vi "Drive Controller.vi"(8 "error in":errorcluster) -> ()   [LabVIEW 2018]
doc: "This VI executes continuously carrying out the current operation and responding to updates or new operation requests. It will often contain the timing or control code that is difficult to place directly in TeleOp. This VI generally opens all sensors and motors and isolates the rest of the robot code from knowing implementation details of how the operations are carried out."
uses:
  Drive Setpoints.ctl
  Drive Operations.ctl
  <vilib>/Rock Robotics/WPI/Solenoid/WPI_SolenoidChannel.ctl
  <vilib>/Rock Robotics/WPI/SafetyOutput/WPI_SafetyOutputConfigMenu.ctl
  <vilib>/Rock Robotics/WPI/ThirdParty/Phoenix-LabVIEW/Motor Controller/Controls/CTRE_Phoenix_MotorControl_NeutralMode.ctl
  <vilib>/Rock Robotics/WPI/ThirdParty/Phoenix-LabVIEW/Motor Controller/Controls/CTRE_Phoenix_MotorControl_FeedbackDevice.ctl
  <vilib>/Rock Robotics/WPI/ThirdParty/Phoenix-LabVIEW/Motor Controller/Controls/CTRE_Phoenix_MotorControl_ControlMode.ctl
  <vilib>/Rock Robotics/WPI/ThirdParty/Phoenix-LabVIEW/Motor Controller/Controls/CTRE_Phoenix_MotorControl_StatusFrameEnhanced.ctl
  <vilib>/Rock Robotics/WPI/Solenoid/WPI_SolenoidValue.ctl
  <vilib>/Rock Robotics/WPI/Solenoid/WPI_SolenoidOpenSingle.vi
  <vilib>/Rock Robotics/WPI/Solenoid/WPI_SolenoidSetEnum.vi
  <vilib>/Rock Robotics/WPI/Utilities/WPI_GetSetVariantRefNum.vi
  <vilib>/Rock Robotics/WPI/RobotDrive/WPI_RobotDriveMecanumDrive_Cartesian.vi
  <vilib>/Rock Robotics/WPI/ThirdParty/Phoenix-LabVIEW/Motor Controller/Get/CTRE_Phoenix_MotorController_GetQuadratureData.vi
panel:
  out "Current\nCmd":string
  # ".578"
  # "Tip: It may be helpful to observe inputs and sensor values.\nYou may also want to display tuning or debugging controls."
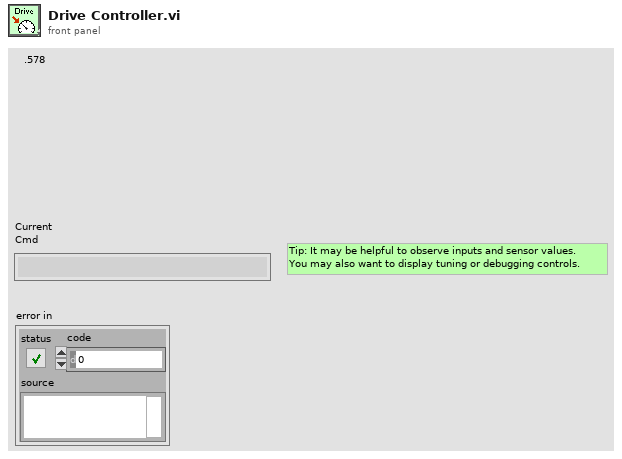
[diagram p1: front panel]
types:
  T1 = typedef "CTRE_Phoenix_MotorControl_StatusFrameEnhanced.ctl" = u16
  T2 = typedef "WPI_SolenoidChannel.ctl" = enum8{"Solenoid 0", "Solenoid 1", "Solenoid 2", "Solenoid 3", "Solenoid 4", "Solenoid 5", "Solenoid 6", "Solenoid 7", "Invalid"}
  T3 = typedef "CTRE_Phoenix_MotorControl_FeedbackDevice.ctl" = i8
  T4 = typedef "CTRE_Phoenix_MotorControl_NeutralMode.ctl" = enum8{"EEPROMSetting", "Override to Coast", "Override to Brake"}
  T5 = typedef "CTRE_Phoenix_MotorControl_ControlMode.ctl" = u16
  T6 = typedef "WPI_SafetyOutputConfigMenu.ctl" = enum16{"Enable", "Disable"}
  T7 = typedef "Drive Setpoints.ctl" = cluster{"Operation":T8, "X Setpoint":dbl, "Y Setpoint":dbl, "Duration":dbl, "Z Setpoint":dbl, "Tracks":bool, "Gyro":dbl, "POV":i16, "Distance(feet)":dbl, "AutoTrack Toggle":bool, "Collsision Detection":bool, "Reset Encoder":bool, "MP File Name":string}
  T8 = typedef "Drive Operations.ctl" = enum16{"Reserve", "Read Current", "Reset Motors VBus", "Motion Profile run", "Immediate Robot Centric", "Drive for Time Robot Centric", "Immediate Field Centric", "Drive For Time Field Centric", "Button Adjust", "Set Motors Motion Profile", "Reset Encoders", "Motion Profile Enable", "Drive for Distance"}
  T9 = typedef "WPI_MotorControlDeviceRef.ctl" = cluster{"DeviceStatus":errorcluster, "Type":T10, "PWM":cluster{"PWM Channel":T11, "DeadBand":T12}, "CAN":cluster{"Device Number":u8, "SetOutput VI Ref":variant, "GetOutput VI Ref":variant, "Enable VI Ref":variant, "Disable VI Ref":variant, "Data":variant}, "Invert":bool, "DIO PWM":cluster{"PWM \"Enable\" Channel":T11, "DIOChannel":T13, "PWM Rate":dbl}}
  T10 = typedef "WPI_MotorControlType.ctl" = enum16{"PWM", "CAN", "DIO PWM"}
  T11 = typedef "FPGA_DIOPWMChannel.ctl" = enum8{"PWM 0", "PWM 1", "PWM 2", "PWM 3", "PWM 4", "PWM 5", "PWM 6", "PWM 7", "PWM 8", "PWM 9", "PWM MXP 0", "PWM MXP 1", "PWM MXP 2", "PWM MXP 3", "PWM MXP 4", "PWM MXP 5", "PWM MXP 6", "PWM MXP 7", "PWM MXP 8", "PWM MXP 9", "Invalid"}
  T12 = typedef "WPI_PWMDeadband.ctl" = cluster{"Name":string, "maxPositivePwm":i32, "minPositivePwm":i32, "centerPwm":i32, "maxNegativePwm":i32, "minNegativePwm":i32, "angularRange":u16}
  T13 = typedef "FPGA_DIOChannel.ctl" = enum8{"DIO 0", "DIO 1", "DIO 2", "DIO 3", "DIO 4", "DIO 5", "DIO 6", "DIO 7", "DIO 8", "DIO 9", "DIO MXP 0", "DIO MXP 1", "DIO MXP 2", "DIO MXP 3", "DIO MXP 4", "DIO MXP 5", "DIO MXP 6", "DIO MXP 7", "DIO MXP 8", "DIO MXP 9", "DIO MXP 10", "DIO MXP 11", "DIO MXP 12", "DIO MXP 13", "DIO MXP 14", "DIO MXP 15", "SPI Port CS1", "SPI Port CS2", "SPI Port CS3", "SPI Port MISO", "SPI Port MOSI", "Invalid"}
  T14 = typedef "WPI_RobotDriveDevRef.ctl" = cluster{"DevStatus":errorcluster, "Motors[]":T9[], "Square Inputs":bool, "Max Output":dbl}
  T15 = typedef "WPI_SolenoidDevRef.ctl" = cluster{"DevStatus":errorcluster, "Pneumatics Control Module":u8, "Forward Solenoid Channel":T2, "Reverse Solenoid Channel":T2}
  T16 = typedef "Command Status Info.ctl" = cluster{"Name":string, "Status":T17, "notifier out":T18}
  T17 = typedef "Completion Status.ctl" = enum16{"Successful", "Aborted", "Incomplete"}
  T18 = typedef "Completion Notifier.ctl" = refnum<notifier>
  T19 = cluster{"SubSystem Data":T7, cluster{"Start Time (ms)":u32, "Iterations":i32}, cluster{"Command Info":T16, "Description":string, "SubSystem Data":T7, "notifier out":refnum<notifier>, "Subsystem Name":string}}
  T20 = cluster{"proportional gain (Kc)":dbl, "integral time (Ti, min)":dbl, "derivative time (Td, min)":dbl}
  T21 = typedef "WPI_SolenoidValue.ctl" = enum16{"Off", "On", "Forward", "Reverse"}
  T22 = cluster{"SubSystem Data":T7, cluster{"Start Time (ms)":u32, "Iterations":i32}, "Default Command Arguments":cluster{"Command Info":T16, "Description":string, "SubSystem Data":T7, "notifier out":refnum<notifier>, "Subsystem Name":string}}
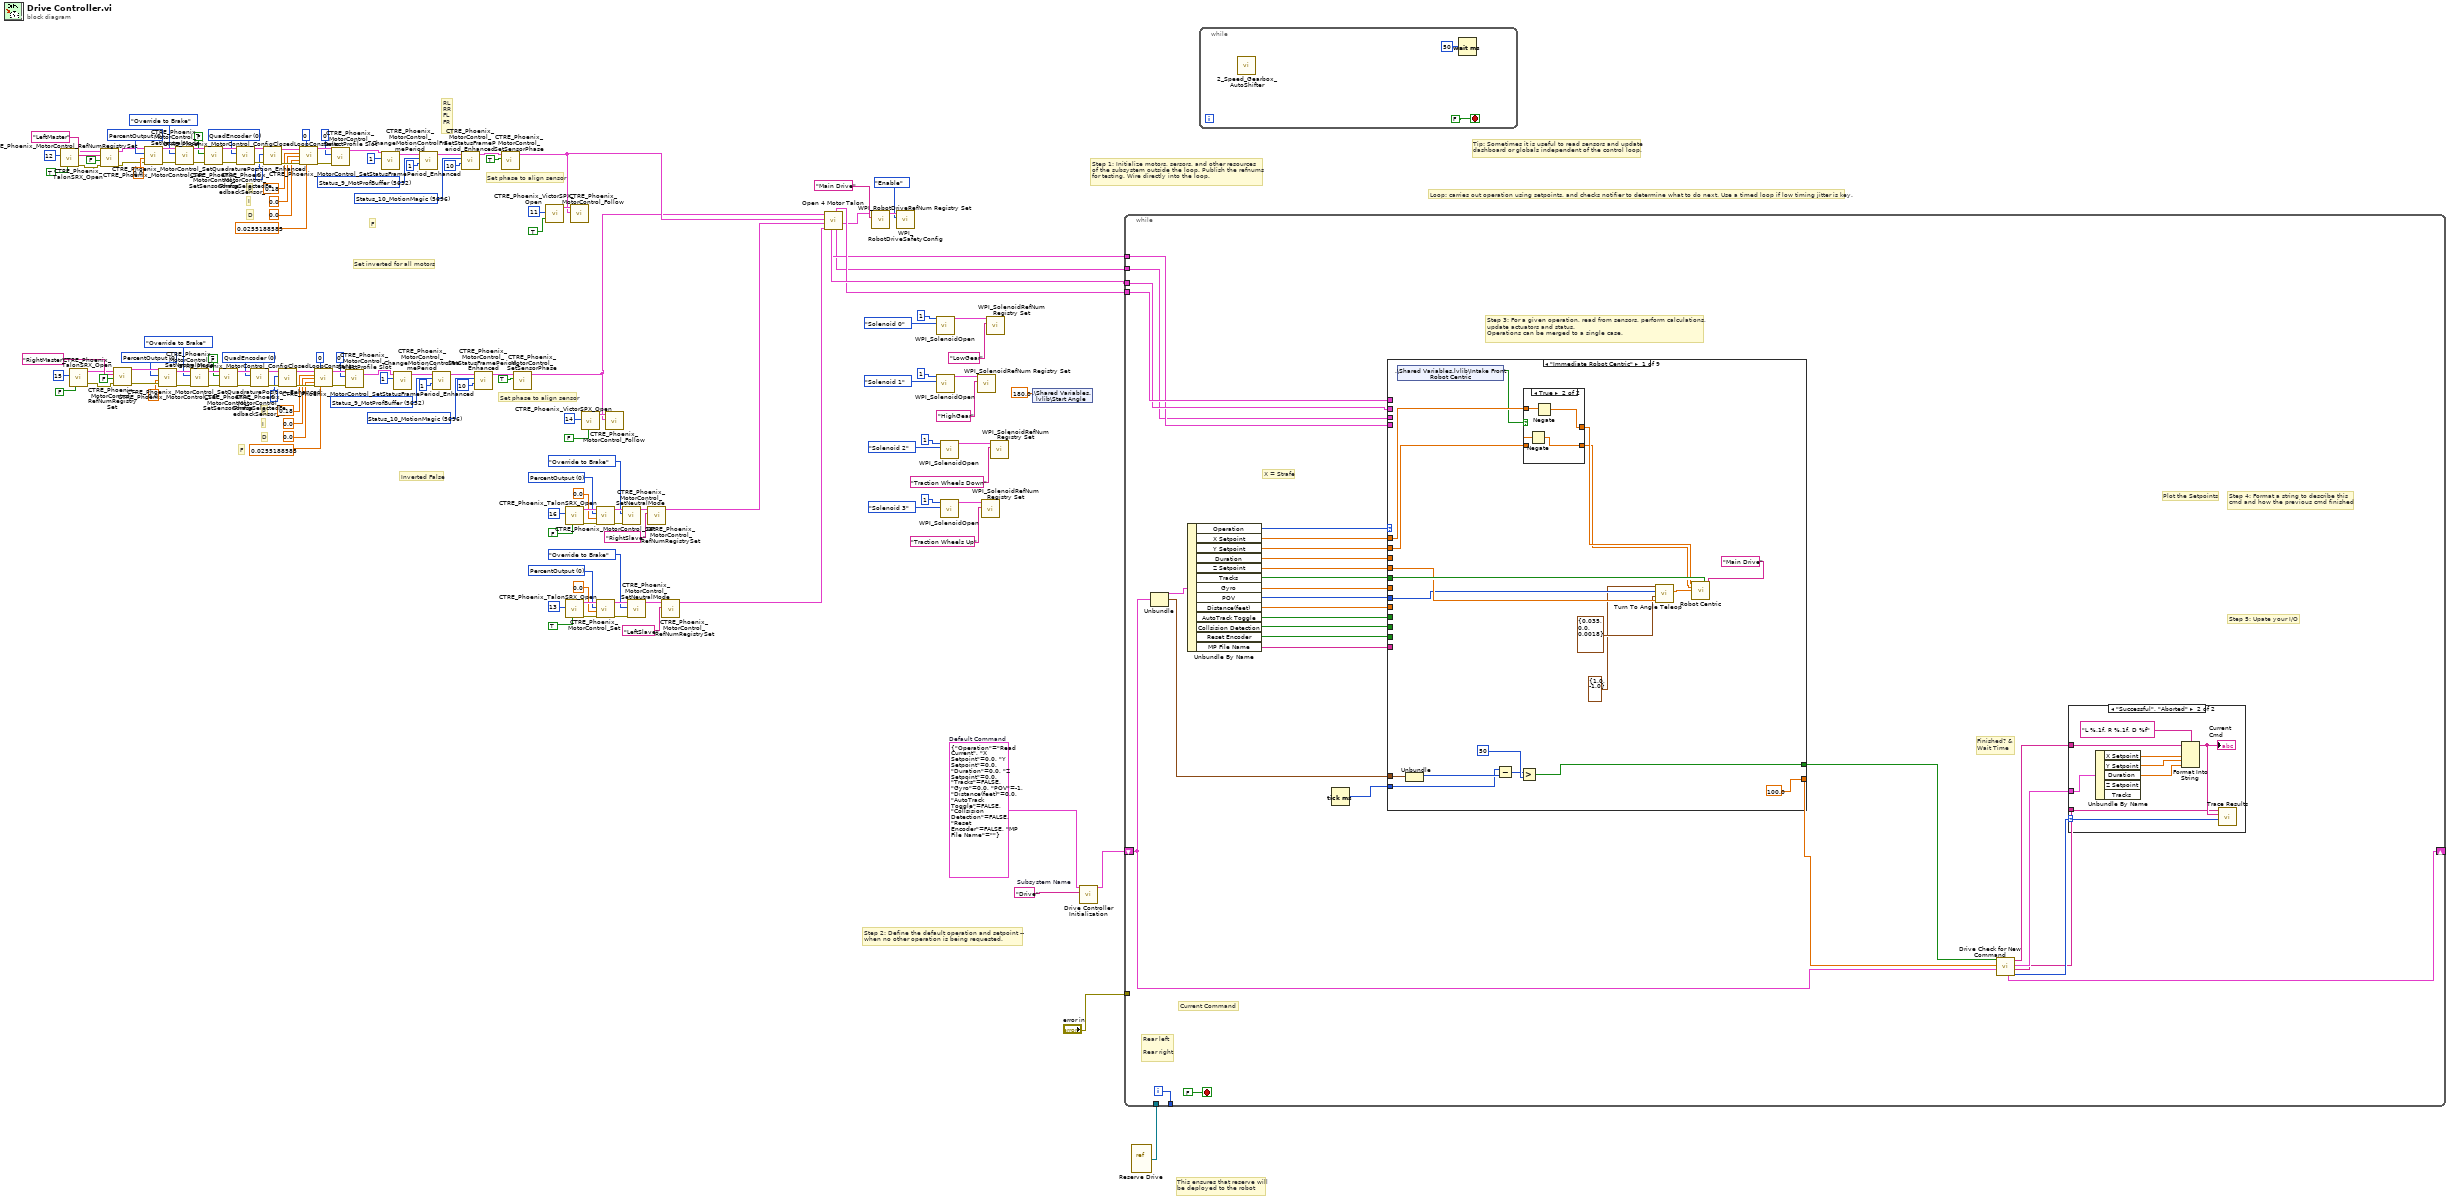
[diagram p0: block diagram]
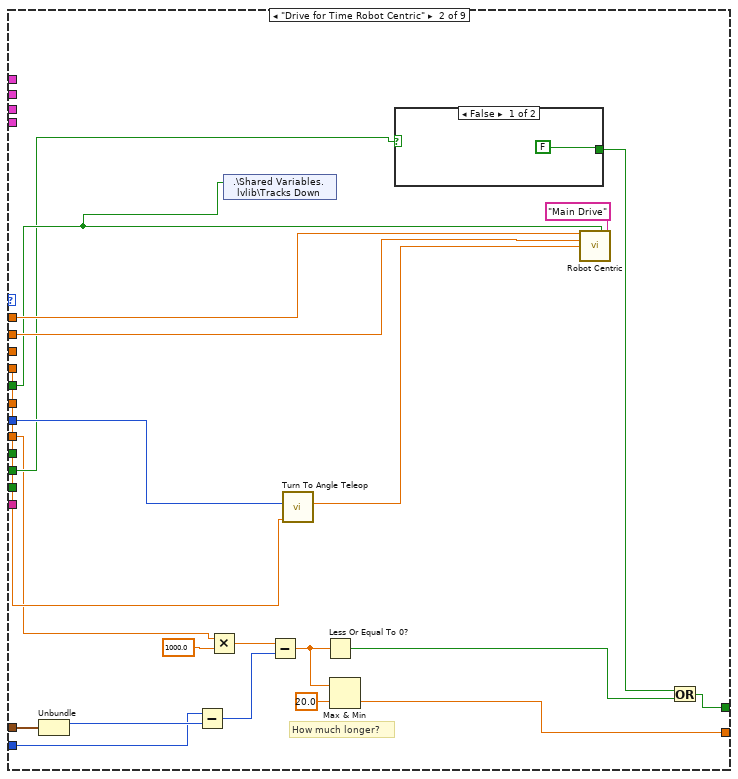
[diagram p4: hidden frame]
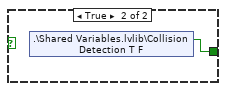
[diagram p5: hidden frame]
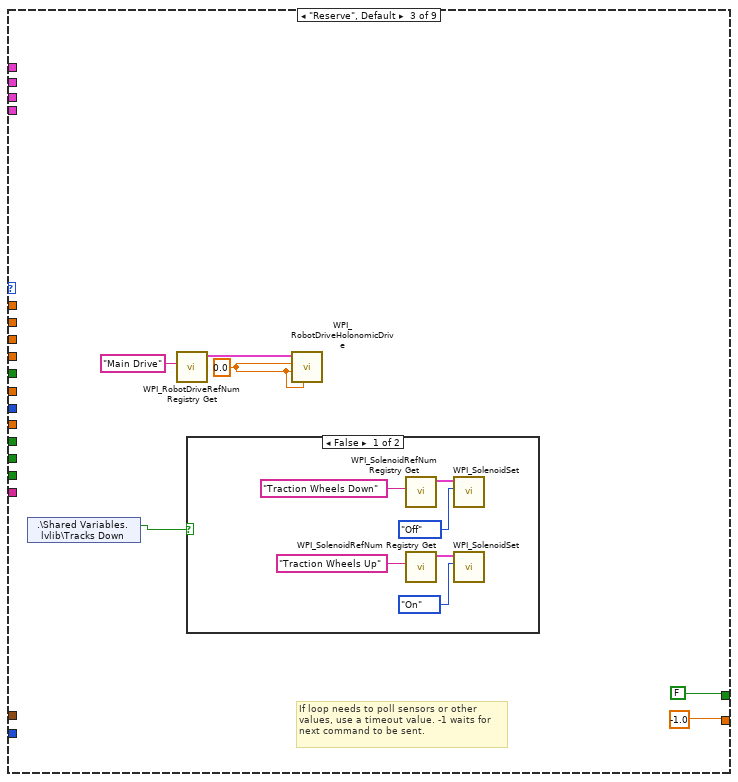
[diagram p6: hidden frame]
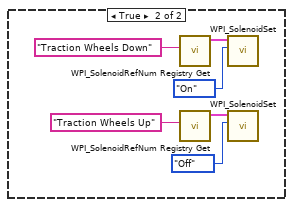
[diagram p7: hidden frame]
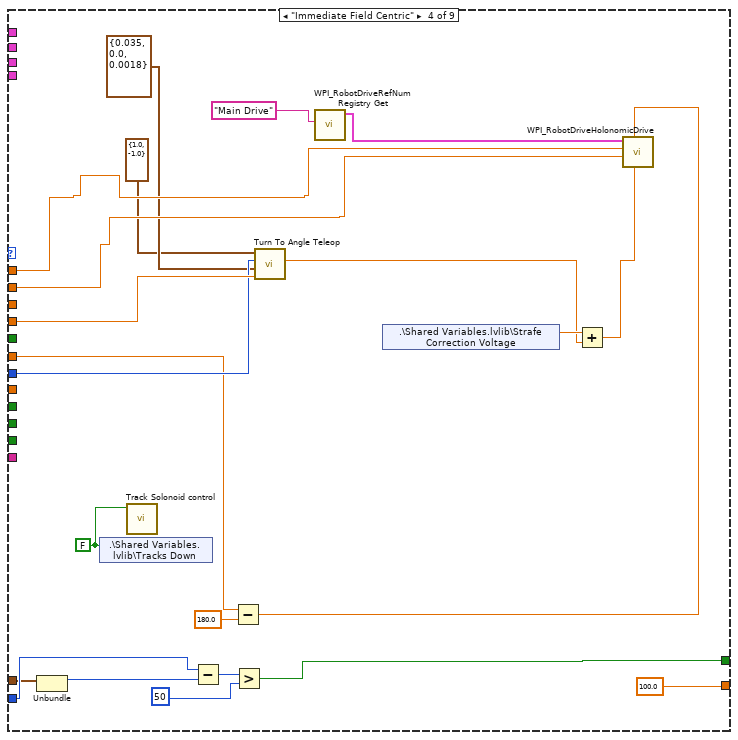
[diagram p8: hidden frame]
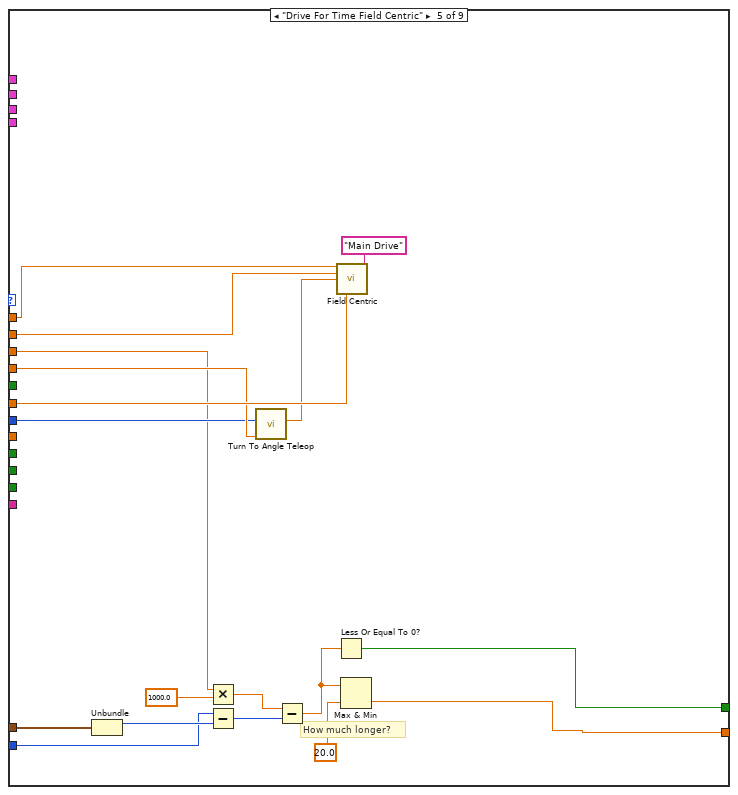
[diagram p9: hidden frame]
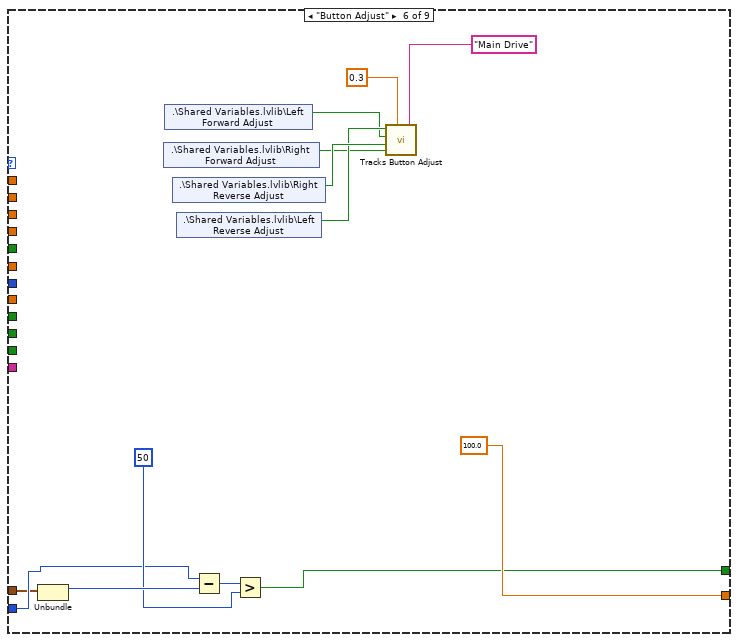
[diagram p10: hidden frame]
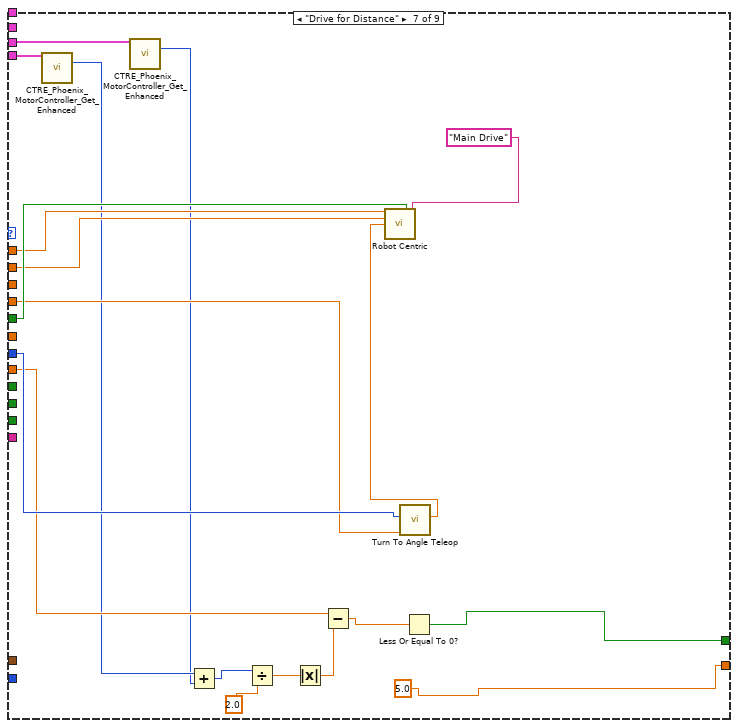
[diagram p11: hidden frame]
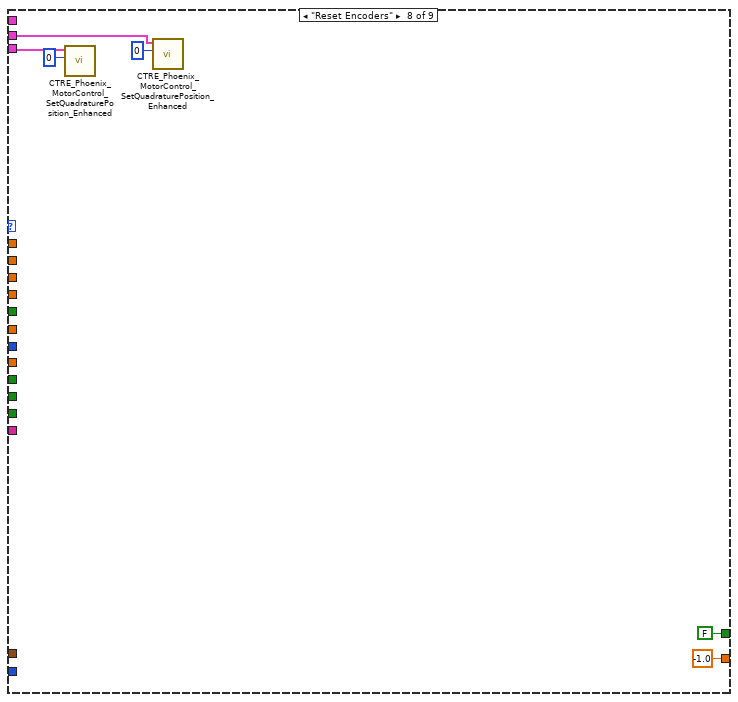
[diagram p12: hidden frame]
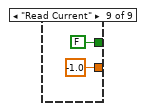
[diagram p13: hidden frame]
diagram:
  w13 = T1 5696 items=["Status_1_General"=5120, "Status_2_Feedback0"=5184, "Status_3_Quadrature"=5248, "Status_4_AinTempVbat"=5312, "Status_6_Misc"=5440, "Status_7_CommStatus"=5504, "Status_8_PulseWidth"=5568, "Status_9_MotProfBuffer"=5632, "Status_10_MotionMagic"=5696, "Status_11_UartGadgeteer"=5760, "Status_12_Feedback1"=5824, "Status_13_Base_PIDF0"=5888, "Status_14_Turn_PIDF1"=5952, "Status_15_FirmwareApiStatus"=6016] ("Status Frame")
  w15 = T1 5632 items=["Status_1_General"=5120, "Status_2_Feedback0"=5184, "Status_3_Quadrature"=5248, "Status_4_AinTempVbat"=5312, "Status_6_Misc"=5440, "Status_7_CommStatus"=5504, "Status_8_PulseWidth"=5568, "Status_9_MotProfBuffer"=5632, "Status_10_MotionMagic"=5696, "Status_11_UartGadgeteer"=5760, "Status_12_Feedback1"=5824, "Status_13_Base_PIDF0"=5888, "Status_14_Turn_PIDF1"=5952, "Status_15_FirmwareApiStatus"=6016] ("Status Frame")
  w24 = T1 5696 items=["Status_1_General"=5120, "Status_2_Feedback0"=5184, "Status_3_Quadrature"=5248, "Status_4_AinTempVbat"=5312, "Status_6_Misc"=5440, "Status_7_CommStatus"=5504, "Status_8_PulseWidth"=5568, "Status_9_MotProfBuffer"=5632, "Status_10_MotionMagic"=5696, "Status_11_UartGadgeteer"=5760, "Status_12_Feedback1"=5824, "Status_13_Base_PIDF0"=5888, "Status_14_Turn_PIDF1"=5952, "Status_15_FirmwareApiStatus"=6016] ("Status Frame")
  w26 = T1 5632 items=["Status_1_General"=5120, "Status_2_Feedback0"=5184, "Status_3_Quadrature"=5248, "Status_4_AinTempVbat"=5312, "Status_6_Misc"=5440, "Status_7_CommStatus"=5504, "Status_8_PulseWidth"=5568, "Status_9_MotProfBuffer"=5632, "Status_10_MotionMagic"=5696, "Status_11_UartGadgeteer"=5760, "Status_12_Feedback1"=5824, "Status_13_Base_PIDF0"=5888, "Status_14_Turn_PIDF1"=5952, "Status_15_FirmwareApiStatus"=6016] ("Status Frame")
  w55 = T3 0 items=["None"=-1, "QuadEncoder"=0, "Analog"=2, "Tachometer"=4, "Pulse Width Encoded Position"=8, "Sensor Sum (S0 + S1)"=9, "Sensor Difference (D0 - D1)"=10, "Remote Source 0"=11, "Remote Source 1"=12, "Software Emulated"=15] ("Feedback Device")
  w38 = T5 0 items=["PercentOutput"=0, "Position"=1, "Velocity"=2, "Current"=3, "Follower"=5, "MotionProfile"=6, "MotionMagic"=7, "MotionMagicArc"=8, "MotionProfileArc"=10, "Disabled"=15] ("Control Mode")
  w84 = T3 0 items=["None"=-1, "QuadEncoder"=0, "Analog"=2, "Tachometer"=4, "Pulse Width Encoded Position"=8, "Sensor Sum (S0 + S1)"=9, "Sensor Difference (D0 - D1)"=10, "Remote Source 0"=11, "Remote Source 1"=12, "Software Emulated"=15] ("Feedback Device")
  w69 = T5 0 items=["PercentOutput"=0, "Position"=1, "Velocity"=2, "Current"=3, "Follower"=5, "MotionProfile"=6, "MotionMagic"=7, "MotionMagicArc"=8, "MotionProfileArc"=10, "Disabled"=15] ("Control Mode")
  w100 = T5 0 items=["PercentOutput"=0, "Position"=1, "Velocity"=2, "Follower"=5, "MotionProfile"=6, "MotionMagic"=7, "MotionMagicArc"=8, "TimedPercentOutput"=9, "Disabled"=15] ("Control Mode")
  w108 = T5 0 items=["PercentOutput"=0, "Position"=1, "Velocity"=2, "Follower"=5, "MotionProfile"=6, "MotionMagic"=7, "MotionMagicArc"=8, "TimedPercentOutput"=9, "Disabled"=15] ("Control Mode")
  w145 = T7 {"Operation"=enum."Read Current", "X Setpoint"=0.0, "Y Setpoint"=0.0, "Duration"=0.0, "Z Setpoint"=0.0, "Tracks"=FALSE, "Gyro"=0.0, "POV"=-1, "Distance(feet)"=0.0, "AutoTrack Toggle"=FALSE, "Collsision Detection"=FALSE, "Reset Encoder"=FALSE, "MP File Name"=""}  # Default Command
  w146 = "Drive"  # Subsystem Name
  # "Set phase to align sensor"
  # "Set phase to align sensor"
  # "F"
  # "D"
  # "I"
  # "P"
  # "F"
  # "D"
  # "I"
  # "P"
  # "Set inverted for all motors"
  # "Inverted False"
  # "RL\nRR\nFL\nFR"
  # "This ensures that reserve will\nbe deployed to the robot"
  # "Tip: Sometimes it is useful to read sensors and update\ndashboard or globals independent of the control loop."
  # "Step 2: Define the default operation and setpoint --\nwhen no other operation is being requested."
  # "Step 1: Initialize motors, sersors, and other resources\nof the subsystem outside the loop. Publish the refnums\nfor testing. Wire directly into the loop."
  # "Loop: carries out operation using setpoints, and checks notifier to determine what to do next. Use a timed loop if low timing jitter is key."
  n1 = call <vilib>:"CTRE_Phoenix_TalonSRX_Open.vi"("Invert"=TRUE, "Device Number"=u8 12) -> ("error out"=w119:errorcluster, "CAN Talon SRX Ref"=w120:T9)  [unwired: 8 in]
  n2 = call <vilib>:"CTRE_Phoenix_TalonSRX_Open.vi"("Invert"=FALSE, "Device Number"=u8 15) -> ("error out"=w117:errorcluster, "CAN Talon SRX Ref"=w118:T9)  [unwired: 8 in]
  n3 = call <vilib>:"CTRE_Phoenix_MotorControl_RefNumRegistrySet.vi"("error in (no error)"=w119, "Test Mode Only"=FALSE, "refnum name"="LeftMaster", "PhoenixMotorControlDevRef"=w120) -> ("error out"=w67:errorcluster, "PhoenixMotorControlDevRef"=w68:T9)  [unwired: 6 in]
  n4 = call <vilib>:"CTRE_Phoenix_MotorControl_RefNumRegistrySet.vi"("error in (no error)"=w117, "Test Mode Only"=FALSE, "refnum name"="RightMaster", "PhoenixMotorControlDevRef"=w118) -> ("error out"=w40:errorcluster, "PhoenixMotorControlDevRef"=w41:T9)  [unwired: 6 in]
  n5 = call <vilib>:"CTRE_Phoenix_MotorControl_Set.vi"("error in (no error)"=w67, "Output"=0.0, "Control Mode"=w69, "PhoenixMotorControlDevRef"=w68) -> ("error out"=w88:errorcluster, "PhoenixMotorControlDevRef"=w92:T9)  [unwired: 6 in]
  n6 = call <vilib>:"CTRE_Phoenix_MotorControl_Set.vi"("error in (no error)"=w40, "Output"=0.0, "Control Mode"=w38, "PhoenixMotorControlDevRef"=w41) -> ("error out"=w59:errorcluster, "PhoenixMotorControlDevRef"=w63:T9)  [unwired: 6 in]
  n7 = call <vilib>:"CTRE_Phoenix_MotorControl_SetNeutralMode.vi"("error in (no error)"=w88, "Motor Control Neutral Mode"=CTRE_Phoenix_MotorControl_NeutralMode."Override to Brake", "PhoenixMotorControlDevRef"=w92) -> ("error out"=w90:errorcluster, "PhoenixMotorControlDevRef"=w89:T9)  [unwired: 7 in]
  n8 = call <vilib>:"CTRE_Phoenix_MotorControl_SetNeutralMode.vi"("error in (no error)"=w59, "Motor Control Neutral Mode"=CTRE_Phoenix_MotorControl_NeutralMode."Override to Brake", "PhoenixMotorControlDevRef"=w63) -> ("error out"=w61:errorcluster, "PhoenixMotorControlDevRef"=w60:T9)  [unwired: 7 in]
  n9 = call <vilib>:"CTRE_Phoenix_MotorControl_SetSensorPhase.vi"("error in (no error)"=w90, "PhaseSensor"=FALSE, "PhoenixMotorControlDevRef"=w89) -> ("error out"=w86:errorcluster, "PhoenixMotorControlDevRef"=w85:T9)  [unwired: 7 in]
  n10 = call <vilib>:"CTRE_Phoenix_MotorControl_SetSensorPhase.vi"("error in (no error)"=w61, "PhaseSensor"=FALSE, "PhoenixMotorControlDevRef"=w60) -> ("error out"=w57:errorcluster, "PhoenixMotorControlDevRef"=w56:T9)  [unwired: 7 in]
  n11 = call <vilib>:"CTRE_Phoenix_MotorControl_ConfigSelectedFeedbackSensor_Enhanced.vi"("error in (no error)"=w86, "Feedback Device"=w84, "PhoenixMotorControlDevRef"=w85) -> ("error out"=w82:errorcluster, "PhoenixMotorControlDevRef"=w83:T9)  [unwired: 7 in]
  n12 = call <vilib>:"CTRE_Phoenix_MotorControl_ConfigSelectedFeedbackSensor_Enhanced.vi"("error in (no error)"=w57, "Feedback Device"=w55, "PhoenixMotorControlDevRef"=w56) -> ("error out"=w53:errorcluster, "PhoenixMotorControlDevRef"=w54:T9)  [unwired: 7 in]
  n13 = call <vilib>:"CTRE_Phoenix_MotorControl_SetQuadraturePosition_Enhanced.vi"("error in (no error)"=w82, "New Position"=0, "PhoenixMotorControlDevRef"=w83) -> ("error out"=w79:errorcluster, "PhoenixMotorControlDevRef"=w80:T9)  [unwired: 7 in]
  n14 = call <vilib>:"CTRE_Phoenix_MotorControl_SetQuadraturePosition_Enhanced.vi"("error in (no error)"=w53, "New Position"=0, "PhoenixMotorControlDevRef"=w54) -> ("error out"=w50:errorcluster, "PhoenixMotorControlDevRef"=w51:T9)  [unwired: 7 in]
  n15 = call <vilib>:"CTRE_Phoenix_MotorControl_ConfigClosedLoopConstants.vi"("PhoenixMotorControlDevRef"=w80, "slotIdx"=0, "P"=0.18, "I"=0.0, "D"=0.0, "error in (no error)"=w79, "F"=0.0255188585) -> ("PhoenixMotorControlDevRef"=w72:T9, "error out"=w73:errorcluster)  [unwired: 7 in]
  n16 = call <vilib>:"CTRE_Phoenix_MotorControl_ConfigClosedLoopConstants.vi"("PhoenixMotorControlDevRef"=w51, "slotIdx"=0, "P"=0.18, "I"=0.0, "D"=0.0, "error in (no error)"=w50, "F"=0.0255188585) -> ("PhoenixMotorControlDevRef"=w43:T9, "error out"=w44:errorcluster)  [unwired: 7 in]
  n17 = call <vilib>:"CTRE_Phoenix_MotorControl_SelectProfile Slot.vi"("error in (no error)"=w73, "slotIdx"=0, "PhoenixMotorControlDevRef"=w72) -> ("PhoenixMotorControlDevRef"=w17:T9)  [unwired: 7 in, 1 out]
  n18 = call <vilib>:"CTRE_Phoenix_MotorControl_SelectProfile Slot.vi"("error in (no error)"=w44, "slotIdx"=0, "PhoenixMotorControlDevRef"=w43) -> ("PhoenixMotorControlDevRef"=w5:T9)  [unwired: 7 in, 1 out]
  n19 = call <vilib>:"CTRE_Phoenix_MotorControl_ChangeMotionControlFramePeriod.vi"("periodMs"=1, "PhoenixMotorControlDevRef"=w17) -> ("PhoenixMotorControlDevRef"=w21:T9)  [unwired: 8 in, 1 out]
  n20 = call <vilib>:"CTRE_Phoenix_MotorControl_ChangeMotionControlFramePeriod.vi"("periodMs"=1, "PhoenixMotorControlDevRef"=w5) -> ("PhoenixMotorControlDevRef"=w10:T9)  [unwired: 8 in, 1 out]
  n21 = call <vilib>:"CTRE_Phoenix_MotorControl_SetStatusFramePeriod_Enhanced.vi"("periodMs"=1, "Status Frame"=w26, "PhoenixMotorControlDevRef"=w21) -> ("PhoenixMotorControlDevRef"=w22:T9)  [unwired: 7 in, 1 out]
  n22 = call <vilib>:"CTRE_Phoenix_MotorControl_SetStatusFramePeriod_Enhanced.vi"("periodMs"=1, "Status Frame"=w15, "PhoenixMotorControlDevRef"=w10) -> ("PhoenixMotorControlDevRef"=w11:T9)  [unwired: 7 in, 1 out]
  n23 = call <vilib>:"CTRE_Phoenix_MotorControl_SetStatusFramePeriod_Enhanced.vi"("periodMs"=10, "Status Frame"=w24, "PhoenixMotorControlDevRef"=w22) -> ("PhoenixMotorControlDevRef"=w18:T9)  [unwired: 7 in, 1 out]
  n24 = call <vilib>:"CTRE_Phoenix_MotorControl_SetStatusFramePeriod_Enhanced.vi"("periodMs"=10, "Status Frame"=w13, "PhoenixMotorControlDevRef"=w11) -> ("PhoenixMotorControlDevRef"=w7:T9)  [unwired: 7 in, 1 out]
  n25 = call <vilib>:"CTRE_Phoenix_MotorControl_SetSensorPhase.vi"("PhaseSensor"=TRUE, "PhoenixMotorControlDevRef"=w18) -> ("PhoenixMotorControlDevRef"=w16:T9)  [unwired: 8 in, 1 out]
  n26 = call <vilib>:"CTRE_Phoenix_MotorControl_SetSensorPhase.vi"("PhaseSensor"=TRUE, "PhoenixMotorControlDevRef"=w7) -> ("PhoenixMotorControlDevRef"=w6:T9)  [unwired: 8 in, 1 out]
  n27 = call <vilib>:"CTRE_Phoenix_VictorSPX_Open.vi"("Invert"=TRUE, "Device Number"=u8 11) -> ("CAN Talon SRX Ref"=w66:T9)  [unwired: 8 in, 1 out]
  n28 = call <vilib>:"CTRE_Phoenix_TalonSRX_Open.vi"("Invert"=FALSE, "Device Number"=u8 16) -> ("error out"=w102:errorcluster, "CAN Talon SRX Ref"=w101:T9)  [unwired: 8 in]
  n29 = call <vilib>:"CTRE_Phoenix_TalonSRX_Open.vi"("Invert"=TRUE, "Device Number"=u8 13) -> ("error out"=w110:errorcluster, "CAN Talon SRX Ref"=w109:T9)  [unwired: 8 in]
  n30 = call <vilib>:"CTRE_Phoenix_MotorControl_Follow.vi"("Master Controller to Follow"=w16, "PhoenixMotorControlDevRef"=w66) -> ()  [unwired: 8 in, 2 out]
  n31 = call <vilib>:"CTRE_Phoenix_VictorSPX_Open.vi"("Invert"=FALSE, "Device Number"=u8 14) -> ("CAN Talon SRX Ref"=w65:T9)  [unwired: 8 in, 1 out]
  n32 = call <vilib>:"CTRE_Phoenix_MotorControl_Set.vi"("error in (no error)"=w102, "Output"=0.0, "Control Mode"=w100, "PhoenixMotorControlDevRef"=w101) -> ("error out"=w97:errorcluster, "PhoenixMotorControlDevRef"=w96:T9)  [unwired: 6 in]
  n33 = call <vilib>:"CTRE_Phoenix_MotorControl_Set.vi"("error in (no error)"=w110, "Output"=0.0, "Control Mode"=w108, "PhoenixMotorControlDevRef"=w109) -> ("error out"=w105:errorcluster, "PhoenixMotorControlDevRef"=w104:T9)  [unwired: 6 in]
  n34 = call <vilib>:"CTRE_Phoenix_MotorControl_Follow.vi"("Master Controller to Follow"=w6, "PhoenixMotorControlDevRef"=w65) -> ()  [unwired: 8 in, 2 out]
  n35 = call <vilib>:"CTRE_Phoenix_MotorControl_SetNeutralMode.vi"("error in (no error)"=w97, "Motor Control Neutral Mode"=CTRE_Phoenix_MotorControl_NeutralMode."Override to Brake", "PhoenixMotorControlDevRef"=w96) -> ("PhoenixMotorControlDevRef"=w2:T9)  [unwired: 7 in, 1 out]
  n36 = call <vilib>:"CTRE_Phoenix_MotorControl_SetNeutralMode.vi"("error in (no error)"=w105, "Motor Control Neutral Mode"=CTRE_Phoenix_MotorControl_NeutralMode."Override to Brake", "PhoenixMotorControlDevRef"=w104) -> ("PhoenixMotorControlDevRef"=w4:T9)  [unwired: 7 in, 1 out]
  n37 = call <vilib>:"CTRE_Phoenix_MotorControl_RefNumRegistrySet.vi"("refnum name"="RightSlave", "PhoenixMotorControlDevRef"=w2) -> ("PhoenixMotorControlDevRef"=w1:T9)  [unwired: 8 in, 1 out]
  n38 = call <vilib>:"CTRE_Phoenix_MotorControl_RefNumRegistrySet.vi"("refnum name"="LeftSlave", "PhoenixMotorControlDevRef"=w4) -> ("PhoenixMotorControlDevRef"=w3:T9)  [unwired: 8 in, 1 out]
  n39 = call "Open 4 Motor Talon.vi"("Front Right"=w3, "Front Left"=w1, "Rear Right"=w16, "Rear Left"=w6) -> ("RobotDriveDevRef"=w113:T14, "Rear Right"=w127:T9, "Front RIght"=w129:T9, "Rear Left"=w128:T9, "Front Left"=w130:T9)  [unwired: 3 in]
  n40 = call <vilib>:"WPI_RobotDriveRefNum Registry Set.vi"("refnum name"="Main Drive", "RobotDriveDevRef"=w113) -> ("RobotDriveDevRef"=w115:T14)  [unwired: 2 in, 7 out]
  n41 = call <vilib>:"WPI_RobotDriveSafetyConfig.vi"("mode"=WPI_SafetyOutputConfigMenu."Enable", "RobotDriveDevRef"=w115) -> ()  [unwired: 8 in, 2 out]
  n42 = call-poly <vilib>:"WPI_SolenoidOpen.vi"("Solenoid Channel"=WPI_SolenoidChannel."Solenoid 0", "Pneumatics Control Module (0)"=u8 1) -> ("SolenoidDevRef"=w30:T15)  [unwired: 8 in, 1 out]
  n43 = call-poly <vilib>:"WPI_SolenoidOpen.vi"("Solenoid Channel"=WPI_SolenoidChannel."Solenoid 1", "Pneumatics Control Module (0)"=u8 1) -> ("SolenoidDevRef"=w32:T15)  [unwired: 8 in, 1 out]
  n44 = call-poly <vilib>:"WPI_SolenoidOpen.vi"("Solenoid Channel"=WPI_SolenoidChannel."Solenoid 2", "Pneumatics Control Module (0)"=u8 1) -> ("SolenoidDevRef"=w135:T15)  [unwired: 8 in, 1 out]
  n45 = call-poly <vilib>:"WPI_SolenoidOpen.vi"("Solenoid Channel"=WPI_SolenoidChannel."Solenoid 3", "Pneumatics Control Module (0)"=u8 1) -> ("SolenoidDevRef"=w138:T15)  [unwired: 8 in, 1 out]
  n46 = call <vilib>:"WPI_SolenoidRefNum Registry Set.vi"("refnum name"="HighGear", "SolenoidDevRef"=w32) -> ()  [unwired: 8 in, 2 out]
  n47 = call <vilib>:"WPI_SolenoidRefNum Registry Set.vi"("refnum name"="Traction Wheels Up", "SolenoidDevRef"=w138) -> ()  [unwired: 8 in, 2 out]
  n48 = call <vilib>:"WPI_SolenoidRefNum Registry Set.vi"("refnum name"="LowGear", "SolenoidDevRef"=w30) -> ()  [unwired: 8 in, 2 out]
  n49 = call <vilib>:"WPI_SolenoidRefNum Registry Set.vi"("refnum name"="Traction Wheels Down", "SolenoidDevRef"=w135) -> ()  [unwired: 8 in, 2 out]
  n50 = shared-variable ".\\Shared Variables.lvlib\\Start Angle"(180.0 ("Start Angle")) -> ()  [unwired: 1 in, 1 out]
  n51 = call "Drive Controller Initialization.vi"("Subsystem Name"=w146, "Default Command"=w145) -> ("output cluster"=w143:T19)  [unwired: 9 in]
  n52 = vi-ref "Reserve Drive.vi"() -> (w142:refnum<vi>)
  n53 = while {
    shift-right: [w170] -> _
    shift-left: w143 -> [w159]
    tunnel: [w175] -> _
    tunnel: "error in" -> [_]
    tunnel: w142 -> [_]
    tunnel: w128 -> [w155]
    tunnel: w127 -> [w154]
    tunnel: w130 -> [w157]
    tunnel: w129 -> [w158]
    i -> [w175]
    stop <- FALSE stop-if-true
    # "X = Strafe"
    # "Rear left \n\nRear right"
    # "Step 5: Upate your I/O"
    # "Step 4: Format a string to describe this\ncmd and how the previous cmd finished"
    # "Current Command"
    # "Plot the Setpoints"
    # "Finished? &\nWait Time"
    # "Step 3: For a given operation, read from sensors, perform calculations,\nupdate actuators and status.\nOperations can be merged to a single case."
    n54 = Unbundle(w159) -> ("SubSystem Data"=w174:T7, w166:cluster{"Start Time (ms)":u32, "Iterations":i32})  [unwired: 1 out]
    n55 = Unbundle By Name(w174) -> ("Operation"=w173:T8, "X Setpoint"=w162:dbl, "Y Setpoint"=w161:dbl, "Duration"=w152:dbl, "Z Setpoint"=w165:dbl, "Tracks"=w160:bool, "Gyro"=w164:dbl, "POV"=w153:i16, "Distance(feet)"=w151:dbl, "AutoTrack Toggle"=w150:bool, "Collsision Detection"=w149:bool, "Reset Encoder"=w147:bool, "MP File Name"=w148:string)
    n56 = Tick Count (ms)() -> (millisecond timer value=w172:u32)
    n57 = case shown="\"Immediate Robot Centric\"" w173 {
      tunnel: [100.0 w224 -1.0 100.0 w282 100.0 5.0 ("y") -1.0 ("y") -1.0 ("y")] -> w163
      tunnel: [w199 w218 FALSE ("ignore previous (F)") w268 w281 w299 w321 FALSE ("ignore previous (F)") FALSE ("ignore previous (F)")] -> w156
      tunnel: w166 -> [w198 w229 _ w269 w284 w297 _ _ _]
      tunnel: w162 -> [w193 w221 _ w257 w279 _ w317 _ _]
      tunnel: w161 -> [w191 w220 _ w261 w291 _ w316 _ _]
      tunnel: w172 -> [w200 w227 _ w270 w283 w298 _ _ _]
      tunnel: w165 -> [w195 w214 _ w266 w276 _ w310 _ _]
      tunnel: w160 -> [w196 w216 _ _ _ _ w318 _ _]
      tunnel: w164 -> [_ _ _ w259 w278 _ _ _ _]
      tunnel: w153 -> [w189 w215 _ w265 w275 _ w312 _ _]
      tunnel: w148 -> [_ _ _ _ _ _ _ _ _]
      tunnel: w158 -> [_ _ _ _ _ _ _ _ _]
      tunnel: w157 -> [_ _ _ _ _ _ _ _ _]
      tunnel: w154 -> [_ _ _ _ _ _ w307 w328 _]
      tunnel: w155 -> [_ _ _ _ _ _ w308 w329 _]
      tunnel: w152 -> [_ _ _ _ w274 _ _ _ _]
      tunnel: w151 -> [_ w211 _ _ _ _ w309 _ _]
      tunnel: w150 -> [_ _ _ _ _ _ _ _ _]
      tunnel: w149 -> [_ w212 _ _ _ _ _ _ _]
      tunnel: w147 -> [_ _ _ _ _ _ _ _ _]
      frame "Immediate Robot Centric" {
        n58 = shared-variable ".\\Shared Variables.lvlib\\Intake Front Robot Centric"() -> (w188:bool)  [unwired: 1 in, 1 out]
        n59 = Unbundle(w198) -> ("Start Time (ms)"=w201:u32)  [unwired: 1 out]
        n60 = Subtract(x=w200, y=w201) -> (x-y=w202:u32)
        n61 = Greater?(x=w202, y=u8 50 ("Left Motor")) -> (0:w199:bool)
        n62 = case shown="True" w188 {
          tunnel: w193 -> [w206 w210]
          tunnel: [w206 w209] -> w192
          tunnel: w191 -> [w205 w208]
          tunnel: [w205 w207] -> w190
          frame False {
          }
          frame True {
            n63 = Negate(x=w208) -> (-x=w207:dbl)
            n64 = Negate(x=w210) -> (-x=w209:dbl)
          }
        }
        n65 = call "Turn To Angle Teleop.vi"("Z Axis"=w195, "PID gains"=T20 {"proportional gain (Kc)"=0.035, "integral time (Ti, min)"=0.0, "derivative time (Td, min)"=0.0018}, "POV"=w189, "output range"=cluster{"output high":dbl, "output low":dbl} {"output high"=1.0, "output low"=-1.0}) -> ("Adjustment Voltage"=w194:dbl)  [unwired: 7 in]
        n66 = call "Robot Centric.vi"("X Axis"=w192, "Tracks Down"=w196, "Drive 1"="Main Drive", "Y Axis"=w190, "Z Axis"=w194) -> ()  [unwired: 11 in]
      }
      frame "Drive for Time Robot Centric" {
        # "How much longer?"
        n67 = Unbundle(w229) -> ("Start Time (ms)"=w228:u32)  [unwired: 1 out]
        n68 = Subtract(x=w227, y=w228) -> (x-y=w222:u32)
        n69 = Multiply(x=w211, y=1000.0) -> (x*y=w231:dbl)
        n70 = shared-variable ".\\Shared Variables.lvlib\\Tracks Down"(w216) -> ()  [unwired: 1 in, 1 out]
        n71 = Subtract(x=w231, y=w222) -> (x-y=w226:dbl)
        n72 = call "Turn To Angle Teleop.vi"("Z Axis"=w214, "POV"=w215) -> ("Adjustment Voltage"=w213:dbl)  [unwired: 9 in]
        n73 = Less Or Equal To 0?(x=w226) -> (x <= 0?=w219:bool)
        n74 = Max & Min(x=w226, y=20.0) -> (min(x,y)=w224:dbl)  [unwired: 1 out]
        n75 = case shown="False" w212 {
          tunnel: [FALSE w233] -> w217
          frame False {
          }
          frame True {
            n76 = shared-variable ".\\Shared Variables.lvlib\\Collision Detection T F"() -> (w233:bool)  [unwired: 1 in, 1 out]
          }
        }
        n77 = call "Robot Centric.vi"("X Axis"=w221, "Tracks Down"=w216, "Drive 1"="Main Drive", "Y Axis"=w220, "Z Axis"=w213) -> ()  [unwired: 11 in]
        n78 = Or(x=w217, y=w219) -> (x .or. y?=w218:bool)
      }
      frame "Reserve", Default {
        w235 = 0.0 ("X")
        # "If loop needs to poll sensors or other\nvalues, use a timeout value. -1 waits for\nnext command to be sent."
        n79 = shared-variable ".\\Shared Variables.lvlib\\Tracks Down"() -> (w234:bool)  [unwired: 1 in, 1 out]
        n80 = call <vilib>:"WPI_RobotDriveRefNum Registry Get.vi"("refnum name"="Main Drive" ("Drive 1")) -> ("RobotDriveDevRef"=w237:T14)  [unwired: 9 in, 1 out]
        n81 = case shown="False" w234 {
          frame False {
            n82 = call <vilib>:"WPI_SolenoidRefNum Registry Get.vi"("refnum name"="Traction Wheels Down") -> ("SolenoidDevRef"=w243:T15)  [unwired: 9 in, 1 out]
            n83 = call <vilib>:"WPI_SolenoidRefNum Registry Get.vi"("refnum name"="Traction Wheels Up") -> ("SolenoidDevRef"=w242:T15)  [unwired: 9 in, 1 out]
            n84 = call-poly <vilib>:"WPI_SolenoidSet.vi"("Value"=WPI_SolenoidValue."Off", "SolenoidDevRef"=w243) -> ()  [unwired: 8 in, 2 out]
            n85 = call-poly <vilib>:"WPI_SolenoidSet.vi"("Value"=WPI_SolenoidValue."On", "SolenoidDevRef"=w242) -> ()  [unwired: 8 in, 2 out]
          }
          frame True {
            n86 = call <vilib>:"WPI_SolenoidRefNum Registry Get.vi"("refnum name"="Traction Wheels Down") -> ("SolenoidDevRef"=w249:T15)  [unwired: 9 in, 1 out]
            n87 = call <vilib>:"WPI_SolenoidRefNum Registry Get.vi"("refnum name"="Traction Wheels Up") -> ("SolenoidDevRef"=w248:T15)  [unwired: 9 in, 1 out]
            n88 = call-poly <vilib>:"WPI_SolenoidSet.vi"("Value"=WPI_SolenoidValue."On", "SolenoidDevRef"=w249) -> ()  [unwired: 8 in, 2 out]
            n89 = call-poly <vilib>:"WPI_SolenoidSet.vi"("Value"=WPI_SolenoidValue."Off", "SolenoidDevRef"=w248) -> ()  [unwired: 8 in, 2 out]
          }
        }
        n90 = call-poly <vilib>:"WPI_RobotDriveHolonomicDrive.vi"("Rotation"=w235, "Y"=w235, "X"=w235, "RobotDriveDevRef"=w237) -> ()  [unwired: 5 in, 3 out]
      }
      frame "Immediate Field Centric" {
        w264 = FALSE ("Tracks Down")
        n91 = Unbundle(w269) -> ("Start Time (ms)"=w271:u32)  [unwired: 1 out]
        n92 = shared-variable ".\\Shared Variables.lvlib\\Tracks Down"(w264) -> ()  [unwired: 1 in, 1 out]
        n93 = call "Track Solonoid control.vi"("Manual Tracks"=w264) -> ()  [unwired: 11 in]
        n94 = Subtract(x=w270, y=w271) -> (x-y=w272:u32)
        n95 = Subtract(x=w259, y=180.0) -> (x-y=w258:dbl)
        n96 = Greater?(x=w272, y=u8 50 ("Left Motor")) -> (0:w268:bool)
        n97 = call "Turn To Angle Teleop.vi"("Z Axis"=w266, "PID gains"=T20 {"proportional gain (Kc)"=0.035, "integral time (Ti, min)"=0.0, "derivative time (Td, min)"=0.0018}, "POV"=w265, "output range"=cluster{"output high":dbl, "output low":dbl} {"output high"=1.0, "output low"=-1.0}) -> ("Adjustment Voltage"=w255:dbl)  [unwired: 7 in]
        n98 = call <vilib>:"WPI_RobotDriveRefNum Registry Get.vi"("refnum name"="Main Drive" ("Drive 1")) -> ("RobotDriveDevRef"=w262:T14)  [unwired: 9 in, 1 out]
        n99 = shared-variable ".\\Shared Variables.lvlib\\Strafe Correction Voltage"() -> (w256:dbl)  [unwired: 1 in, 1 out]
        n100 = Add(x=w256, y=w255) -> (x+y=w254:dbl)
        n101 = call-poly <vilib>:"WPI_RobotDriveHolonomicDrive.vi"("Rotation"=w254, "Gyro Angle"=w258, "Y"=w261, "X"=w257, "RobotDriveDevRef"=w262) -> ()  [unwired: 4 in, 3 out]
      }
      frame "Drive For Time Field Centric" {
        # "How much longer?"
        n102 = Unbundle(w284) -> ("Start Time (ms)"=w287:u32)  [unwired: 1 out]
        n103 = Multiply(x=w274, y=1000.0) -> (x*y=w280:dbl)
        n104 = Subtract(x=w283, y=w287) -> (x-y=w289:u32)
        n105 = call "Turn To Angle Teleop.vi"("Z Axis"=w276, "POV"=w275) -> ("Adjustment Voltage"=w277:dbl)  [unwired: 9 in]
        n106 = Subtract(x=w280, y=w289) -> (x-y=w286:dbl)
        n107 = Less Or Equal To 0?(x=w286) -> (x <= 0?=w281:bool)
        n108 = call "Field Centric.vi"("X Axis"=w279, "Drive 1"="Main Drive", "Y Axis"=w291, "Z Axis"=w277, "Gyro"=w278) -> ()  [unwired: 11 in]
        n109 = Max & Min(x=w286, y=20.0) -> (min(x,y)=w282:dbl)  [unwired: 1 out]
      }
      frame "Button Adjust" {
        n110 = Unbundle(w297) -> ("Start Time (ms)"=w303:u32)  [unwired: 1 out]
        n111 = shared-variable ".\\Shared Variables.lvlib\\Right Forward Adjust"() -> (w293:bool)  [unwired: 1 in, 1 out]
        n112 = shared-variable ".\\Shared Variables.lvlib\\Left Forward Adjust"() -> (w292:bool)  [unwired: 1 in, 1 out]
        n113 = shared-variable ".\\Shared Variables.lvlib\\Right Reverse Adjust"() -> (w295:bool)  [unwired: 1 in, 1 out]
        n114 = shared-variable ".\\Shared Variables.lvlib\\Left Reverse Adjust"() -> (w294:bool)  [unwired: 1 in, 1 out]
        n115 = Subtract(x=w298, y=w303) -> (x-y=w302:u32)
        n116 = Greater?(x=w302, y=u8 50 ("Left Motor")) -> (0:w299:bool)
        n117 = call "Tracks Button Adjust.vi"("Left Forward Adjust"=w294, "Left Reverse Adjust"=w292, "Right Forward Adjust"=w295, "Right Reverse Adjust"=w293, "Adjust Speed"=0.3, "Drive 1"="Main Drive") -> ()  [unwired: 1 in]
      }
      frame "Drive for Distance" {
        n118 = call-poly <vilib>:"CTRE_Phoenix_MotorController_Get_Enhanced.vi"("PhoenixMotorControlDevRef"=w308) -> ("Quadrature Position"=w306:i32)  [unwired: 11 in, 3 out]
        n119 = call-poly <vilib>:"CTRE_Phoenix_MotorController_Get_Enhanced.vi"("PhoenixMotorControlDevRef"=w307) -> ("Quadrature Position"=w305:i32)  [unwired: 11 in, 3 out]
        n120 = Add(x=w306, y=w305) -> (x+y=w323:i32)
        n121 = Divide(x=w323, y=2.0) -> (x/y=w320:dbl)
        n122 = Absolute Value(x=w320) -> (abs(x)=w319:dbl)
        n123 = Subtract(x=w309, y=w319) -> (x-y=w314:dbl)
        n124 = call "Turn To Angle Teleop.vi"("Z Axis"=w310, "POV"=w312) -> ("Adjustment Voltage"=w311:dbl)  [unwired: 9 in]
        n125 = call "Robot Centric.vi"("X Axis"=w317, "Tracks Down"=w318, "Drive 1"="Main Drive", "Y Axis"=w316, "Z Axis"=w311) -> ()  [unwired: 11 in]
        n126 = Less Or Equal To 0?(x=w314) -> (x <= 0?=w321:bool)
      }
      frame "Reset Encoders" {
        n127 = call <vilib>:"CTRE_Phoenix_MotorControl_SetQuadraturePosition_Enhanced.vi"("New Position"=0, "PhoenixMotorControlDevRef"=w329) -> ()  [unwired: 8 in, 2 out]
        n128 = call <vilib>:"CTRE_Phoenix_MotorControl_SetQuadraturePosition_Enhanced.vi"("New Position"=0, "PhoenixMotorControlDevRef"=w328) -> ()  [unwired: 8 in, 2 out]
      }
      frame "Read Current" {
      }
    }
    n129 = call "Drive Check for New Command.vi"("input cluster"=w159, "Wait time (ms)"=w163, "Finished?"=w156) -> ("Completion"=w171:T17, "Subsystem Name"=w167:string, "SetPoint"=w168:T7, "Initial Trace String"=w169:string, "output cluster"=w170:T22)  [unwired: 4 in]
    n130 = case shown="\"Successful\", \"Aborted\"" w171 {
      selector: w171 -> [_ w185]
      tunnel: w169 -> [_ w180]
      tunnel: w168 -> [_ w181]
      tunnel: w167 -> [_ w177]
      frame "Incomplete", Default {
        # "Continuing current command"
      }
      frame "Successful", "Aborted" {
        # "Report and setup for next command"
        n131 = Unbundle By Name(w181) -> ("X Setpoint"=w183:dbl, "Y Setpoint"=w184:dbl, "Duration"=w178:dbl)  [unwired: 2 out]
        n132 = Format Into String(format string="L %.1f, R %.1f, D %f", initial string=w180, w183, w184, w178) -> (resulting string=w179:string)  [unwired: 1 in, 1 out]
        "Current\nCmd" <- w179
        n133 = call <vilib>:"Trace Results.vi"("Status of previous command"=w185, "Description"=w179, "Subsystem"=w177) -> ()  [unwired: 9 in]
      }
    }
  }
  n134 = while {
    stop <- FALSE stop-if-true
    n135 = call "2_Speed_Gearbox_AutoShifter.vi"() -> ()  [unwired: 12 in]
    n136 = Wait (ms)(milliseconds to wait=u32 50) -> ()  [unwired: 1 out]
  }
